vi "time in Gamma - PID - V2.vi"(4 "resonance index":i32, 6 "nonzero temperature":dbl=300.0, 8 "adaptive sweep settings":T1={"time gap (min) "=0.0, "Bypass error dialog"=TRUE, "range factor"=1.05, "min gamma(kHz)"=0.005, "max step(Hz)"=1.05, "min step(Hz)"=0.005, "save freq units"=enum."Hz", "Zero signal?"=FALSE, "time in Gamma --OK"=FALSE, "scan mode"=enum."predictive", "power control mode "=enum."power vs Temp", "time-in-gamma mode"=enum."same for all"}, 10 "sweep folder path":path, 11 "Fast sweep settings":T4={"Update rate (Hz)"=250.0, "Start F, Hz"=300000.0, "Stop F"=3500000.0, "Number of points"=23000, "Amplitude"=0.2, "Init&amplitude"=TRUE, "IF"=1000.0, "Time constant"=0.001} {"IF" format="%#_6p"; "Amplitude" min=0.0 max=2.5; "Number of points" format="%.0p"; "Stop F" format="%#_6p"; "Start F, Hz" format="%#_6p"; "Update rate (Hz)" format="%0.2f"}) -> (0 "adaptive sweep settings OUT":T1={"time gap (min) "=0.0, "Bypass error dialog"=TRUE, "range factor"=1.05, "min gamma(kHz)"=0.005, "max step(Hz)"=1.05, "min step(Hz)"=0.005, "save freq units"=enum."Hz", "Zero signal?"=FALSE, "time in Gamma --OK"=FALSE, "scan mode"=enum."predictive", "power control mode "=enum."power vs Temp", "time-in-gamma mode"=enum."same for all"}, 1 "frequencies":dbl[](array[numeric]), 2 "temperatures":dbl[](array[numeric]), 3 "Fast sweep settings out":T4={"Update rate (Hz)"=250.0, "Start F, Hz"=200000.0, "Stop F"=1700000.0, "Number of points"=30000, "Amplitude"=2.1, "Init&amplitude"=TRUE, "IF"=1000.0, "Time constant"=0.1} {"IF" format="%#_6p"; "Amplitude" min=0.0 max=2.5; "Number of points" format="%.0p"; "Stop F" format="%#_6p"; "Start F, Hz" format="%#_6p"; "Update rate (Hz)" format="%0.2f"})   [LabVIEW 2015]
uses:
  Libraries/RUS/Controls/Sweep settings.ctl
  adaptive sweep UI controls.ctl
  next chunk -- algorithm.ctl
  time in gamma mode control.ctl
  ctl -- name dispatcher -- action.ctl
  next chunk - read-write freq PID file - atomic actions .vi
  ctl -- name dispatcher.vi
  Q - not nan -- real.vi
  file -- 9w path.vi
  array -- find index - real.vi
  array -- interpolate -- i.vi
  <vilib>/Utility/libraryn.llb/Check if File or Folder Exists.vi
  file -- read list of lines.vi
  parse -- find first line.vi
  parse -- get list of matches -- numbers.vi
  <vilib>/Utility/file.llb/Write To Spreadsheet File.vi
  <vilib>/Utility/file.llb/Write To Spreadsheet File (string).vi
  <vilib>/gmath/function.llb/Binomial Coefficient.vi
panel:
  out "time in gamma":dbl
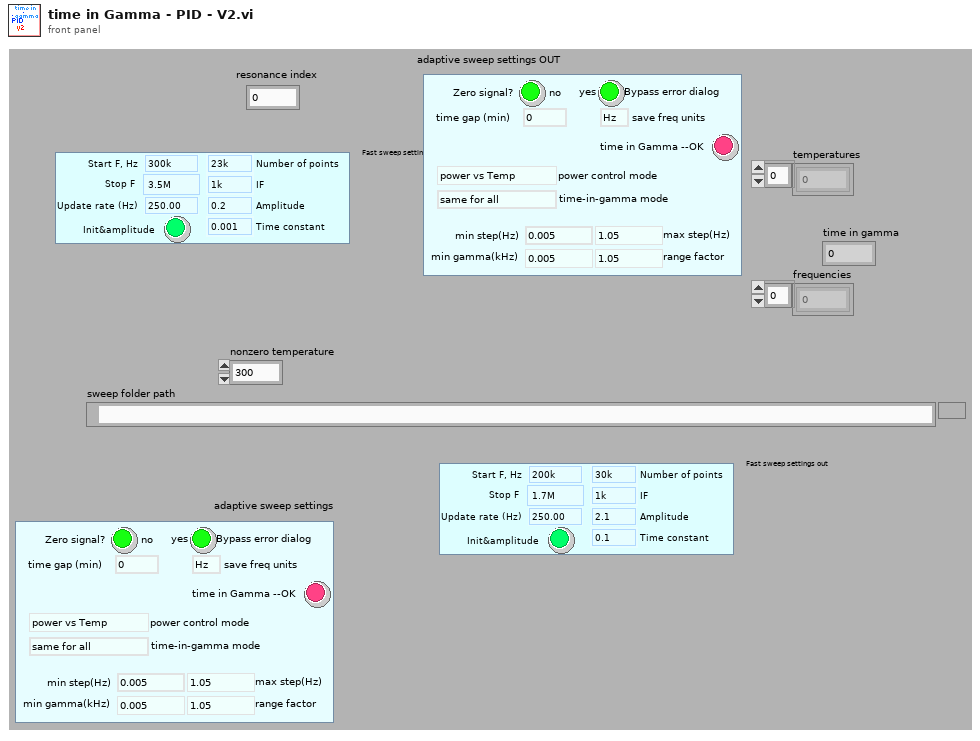
[diagram p1: front panel]
types:
  T1 = typedef "adaptive sweep UI controls.ctl" = cluster{"time gap (min) ":dbl, "Bypass error dialog":bool, "range factor":dbl, "min gamma(kHz)":dbl, "max step(Hz)":dbl, "min step(Hz)":dbl, "save freq units":enum16{"kHz", "Hz"}, "Zero signal?":bool, "time in Gamma --OK":bool, "scan mode":T2, "power control mode ":enum16{"power vs Temp", "power vs Time", "none"}, "time-in-gamma mode":T3}
  T2 = typedef "next chunk -- algorithm.ctl" = enum16{"peak position is known", "uniform", "predictive"}
  T3 = typedef "time in gamma mode control.ctl" = enum16{"same for all", "each one different", "uniform scan"}
  T4 = typedef "Sweep settings.ctl" = cluster{"Update rate (Hz)":dbl, "Start F, Hz":dbl, "Stop F":dbl, "Number of points":i32, "Amplitude":dbl, "Init&amplitude":bool, "IF":dbl, "Time constant":dbl}
  T5 = typedef "ctl -- name dispatcher -- action.ctl" = enum16{"peak frequency", "peak frequency DUMP", "peak gamma DUMP", "peak gamma", "peak frequency TEST", "peak gamma TEST", "ultrasonic power", "time in gamma", "set temperature ", "set temperature timer", "peak default gamma", "last scan file", "peak freq gamma TEST", "peak NAMES", "errors", "P_I_D", "P", "I", "D", "power vs time", "power vs time TIMER", "void", "power log", "set temperature - SINE", "itc ltc log", "peak - time in gamma"}
  T6 = enum16{"same for all", "each one different", "uniform scan"}
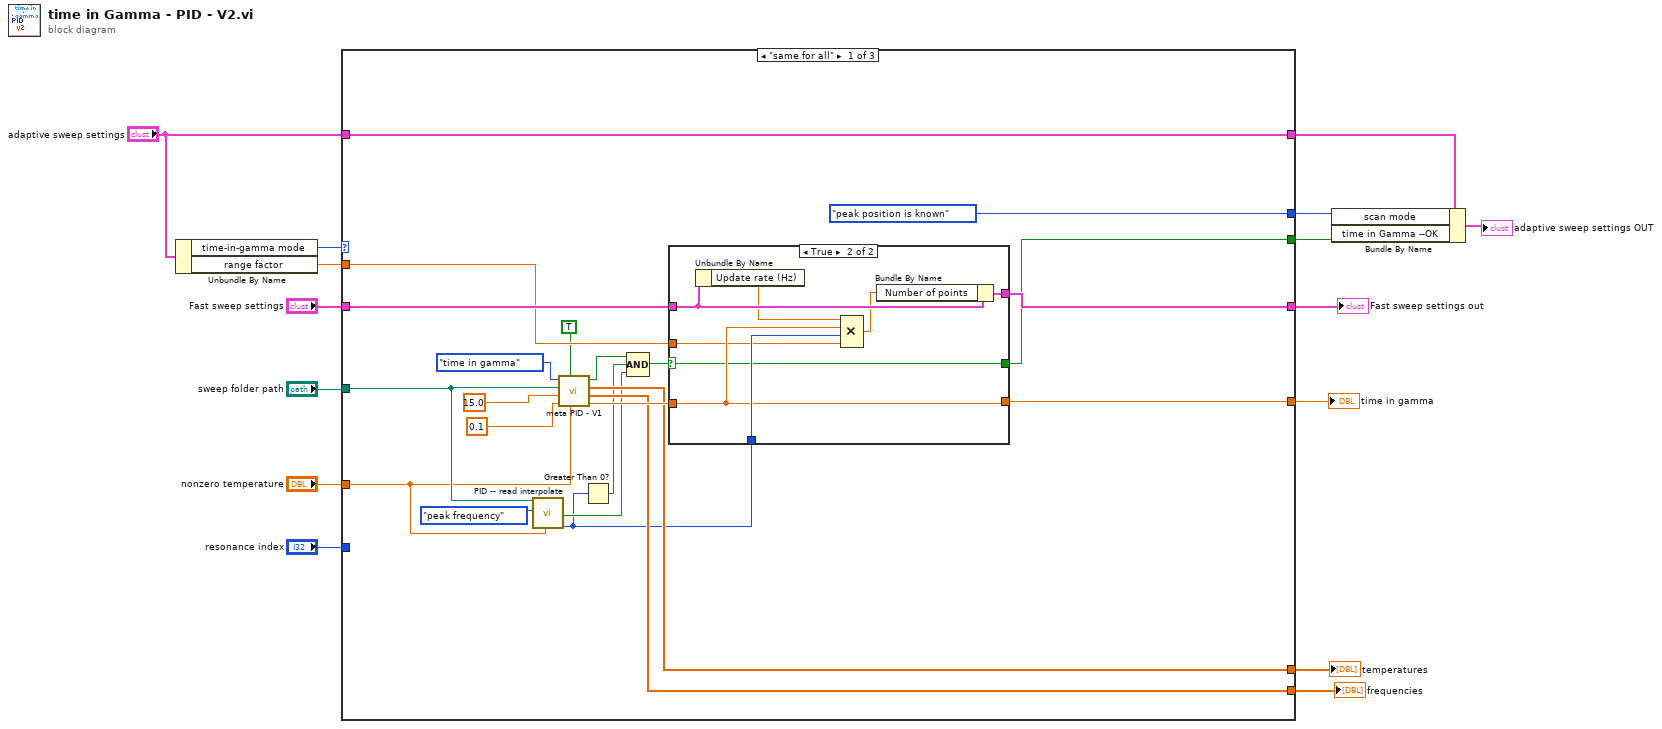
[diagram p0: block diagram]
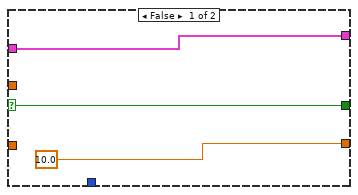
[diagram p2: hidden frame]
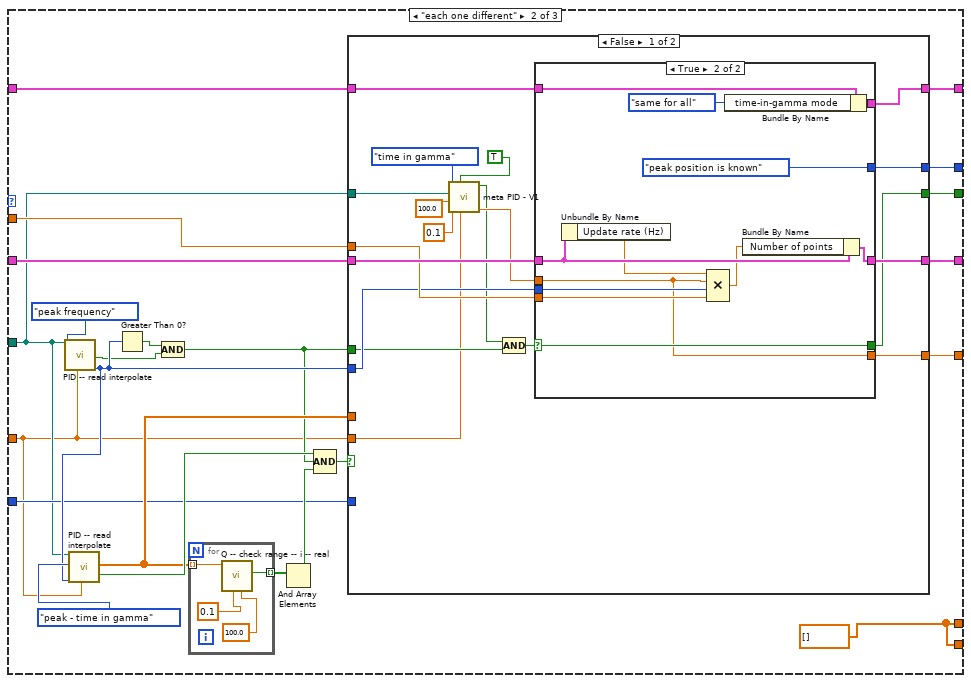
[diagram p3: hidden frame]
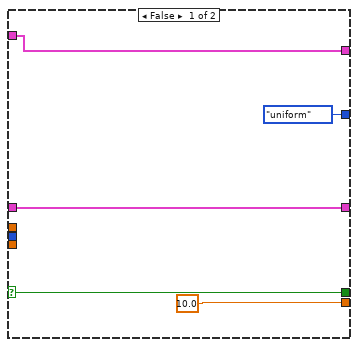
[diagram p4: hidden frame]
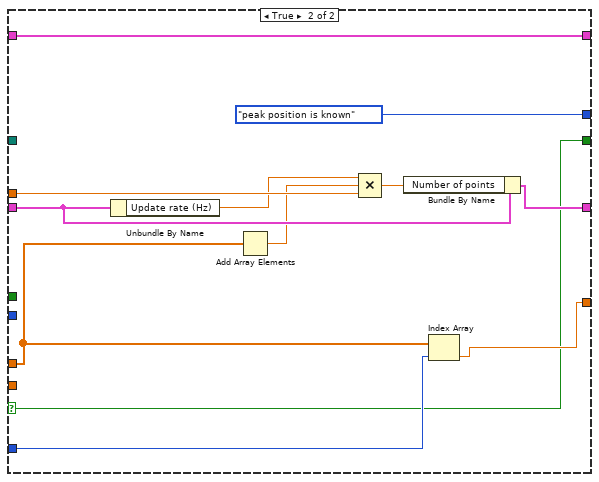
[diagram p5: hidden frame]
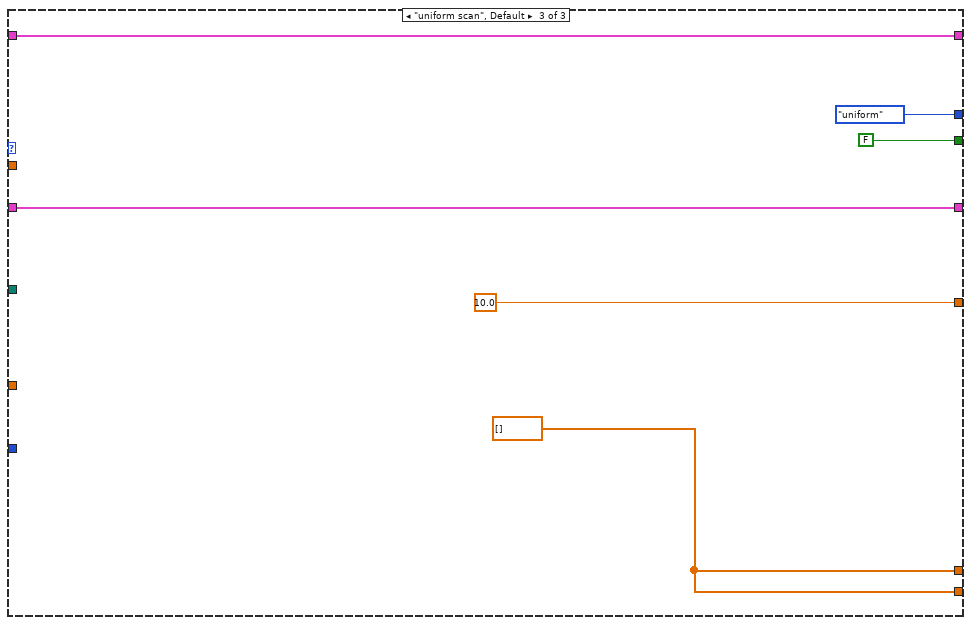
[diagram p6: hidden frame]
diagram:
  n1 = Unbundle By Name("adaptive sweep settings") -> ("time-in-gamma mode"=w8:T3, "range factor"=w5:dbl)
  n2 = case shown="\"same for all\"" w8 {
    tunnel: "Fast sweep settings" -> [w31 w70 w129]
    tunnel: "sweep folder path" -> [w29 w53 _]
    tunnel: "nonzero temperature" -> [w28 w52 _]
    tunnel: [w30 w69 w129] -> w12
    tunnel: [w37 w71 10.0 ("upper")] -> w11
    tunnel: [w32 w49 w127] -> w10
    tunnel: [w33 w49 w127] -> w9
    tunnel: [w20 w67 FALSE] -> w7
    tunnel: w5 -> [w19 w66 _]
    tunnel: [next_chunk_--_algorithm."peak position is known" ("next chunk algorithm") w65 next_chunk_--_algorithm."uniform" ("next chunk algorithm")] -> w4
    tunnel: "resonance index" -> [_ w57 _]
    tunnel: "adaptive sweep settings" -> [w17 w51 w124]
    tunnel: [w17 w50 w124] -> w1
    frame "same for all" {
      n3 = call "PID -- read interpolate.vi"("sweep folder path"=w29, "ctl PID file IN"=ctl_--_name_dispatcher_--_action."peak frequency", "temperature"=w28) -> ("PID OK !"=w24:bool, "length out"=w23:i32)  [unwired: 11 in, 4 out]
      n4 = call "meta PID - V1.vi"("input parameter"=w28, "control?"=TRUE, "lower limit"=0.1 ("lower"), "upper limit"=15.0 ("upper"), "sweep folder path"=w29, "ctl name dispatch"=ctl_--_name_dispatcher_--_action."time in gamma") -> ("bezier output"=w34:dbl, "frequencies"=w33:dbl[], "temperatures"=w32:dbl[], "ok"=w26:bool)  [unwired: 2 in]
      n5 = Greater Than 0?(x=w23) -> (x > 0?=w27:bool)
      n6 = Compound Arithmetic op=AND(w26, w27, w24) -> (w25:bool)
      n7 = case shown="True" w25 {
        selector: w25 -> [w38 w42]
        tunnel: [w39 w48] -> w30
        tunnel: [10.0 ("upper") w46] -> w37
        tunnel: w34 -> [_ w46]
        tunnel: w31 -> [w39 w45]
        tunnel: w23 -> [_ w47]
        tunnel: [w38 w42] -> w20
        tunnel: w19 -> [_ w41]
        frame False {
        }
        frame True {
          n8 = Unbundle By Name(w45) -> ("Update rate (Hz)"=w44:dbl)
          n9 = Compound Arithmetic op=MULTIPLY(w44, w46, w47, w41) -> (w43:dbl)
          n10 = Bundle By Name(cluster=w45, "Number of points"=w43) -> (w48:T4)
        }
      }
    }
    frame "each one different" {
      w49 = dbl[] [] ("temperatures")
      n11 = call "PID -- read interpolate.vi"("sweep folder path"=w53, "ctl PID file IN"=ctl_--_name_dispatcher_--_action."peak frequency", "temperature"=w52) -> ("PID OK !"=w55:bool, "length out"=w63:i32)  [unwired: 11 in, 4 out]
      n12 = call "PID -- read interpolate.vi"("sweep folder path"=w53, "ctl PID file IN"=ctl_--_name_dispatcher_--_action."peak - time in gamma", "length"=w63, "temperature"=w52) -> ("PID freq"=w58:dbl[], "Length OK !"=w62:bool)  [unwired: 10 in, 4 out]
      n13 = Greater Than 0?(x=w63) -> (x > 0?=w56:bool)
      n14 = Compound Arithmetic op=AND(w56, w55) -> (w54:bool)
      n15 = for {
        tunnel: w58 -> [w123] mode=indexing
        tunnel: [w120] -> w61 mode=indexing
        n16 = call "Q -- check range -- i -- real.vi"("upper"=100.0, "lower"=0.1, "number"=w123) -> ("in range?"=w120:bool)  [unwired: 6 in, 2 out]
      }
      n17 = And Array Elements(Boolean array=w61) -> (logical AND=w60:bool)
      n18 = Compound Arithmetic op=AND(w62, w54, w60) -> (w59:bool)
      n19 = case shown="False" w59 {
        selector: w59 -> [_ w109]
        tunnel: [w90 w110] -> w71
        tunnel: w70 -> [w89 w119]
        tunnel: [w88 w118] -> w69
        tunnel: [w87 w109] -> w67
        tunnel: w66 -> [w86 w117]
        tunnel: [w80 next_chunk_--_algorithm."peak position is known" ("next chunk algorithm")] -> w65
        tunnel: w63 -> [w85 _]
        tunnel: w58 -> [_ w112]
        tunnel: w57 -> [_ w111]
        tunnel: w54 -> [w79 _]
        tunnel: w53 -> [w76 _]
        tunnel: w52 -> [w75 _]
        tunnel: w51 -> [w73 w108]
        tunnel: [w72 w108] -> w50
        frame False {
          n20 = call "meta PID - V1.vi"("input parameter"=w75, "control?"=TRUE, "lower limit"=0.1 ("lower"), "upper limit"=100.0 ("upper"), "sweep folder path"=w76, "ctl name dispatch"=ctl_--_name_dispatcher_--_action."time in gamma") -> ("bezier output"=w81:dbl, "ok"=w78:bool)  [unwired: 2 in, 2 out]
          n21 = Compound Arithmetic op=AND(w78, w79) -> (w74:bool)
          n22 = case shown="True" w74 {
            selector: w74 -> [w93 w102]
            tunnel: [w94 w107] -> w88
            tunnel: [10.0 ("upper") w100] -> w90
            tunnel: w89 -> [w94 w105]
            tunnel: w85 -> [_ w106]
            tunnel: [w93 w102] -> w87
            tunnel: w86 -> [_ w101]
            tunnel: w81 -> [_ w100]
            tunnel: [next_chunk_--_algorithm."uniform" ("next chunk algorithm") next_chunk_--_algorithm."peak position is known" ("next chunk algorithm")] -> w80
            tunnel: w73 -> [w91 w98]
            tunnel: [w91 w96] -> w72
            frame False {
            }
            frame True {
              n23 = Unbundle By Name(w105) -> ("Update rate (Hz)"=w104:dbl)
              n24 = Compound Arithmetic op=MULTIPLY(w104, w100, w106, w101) -> (w103:dbl)
              n25 = Bundle By Name(cluster=w98, "time-in-gamma mode"=T6."same for all") -> (w96:T1)
              n26 = Bundle By Name(cluster=w105, "Number of points"=w103) -> (w107:T4)
            }
          }
        }
        frame True {
          n27 = Unbundle By Name(w119) -> ("Update rate (Hz)"=w115:dbl)
          n28 = Add Array Elements(numeric array=w112) -> (sum=w113:dbl)
          n29 = Compound Arithmetic op=MULTIPLY(w115, w113, w117) -> (w114:dbl)
          n30 = Bundle By Name(cluster=w119, "Number of points"=w114) -> (w118:T4)
          n31 = Index Array(array=w112, index=w111) -> (element=w110:dbl)
        }
      }
    }
    frame "uniform scan", Default {
      w127 = dbl[] [] ("temperatures")
    }
  }
  "Fast sweep settings out" <- w12
  "time in gamma" <- w11
  "temperatures" <- w10
  "frequencies" <- w9
  n32 = Bundle By Name(cluster=w1, "scan mode"=w4, "time in Gamma --OK"=w7) -> (→"adaptive sweep settings OUT":T1)
